vi "ModRegistered.vi"(8 "error in (no error)":errorcluster, 11 "JQMHStartup in":refnum<class "RQMHStartup.lvclass">) -> (0 "error out":errorcluster)   [LabVIEW 2024, in "RQMHStartup.lvclass"]
uses:
  RQMHStartup.lvclass
  Command.ctl
  RQMHStartup.lvclass/RQMHStartup.ctl
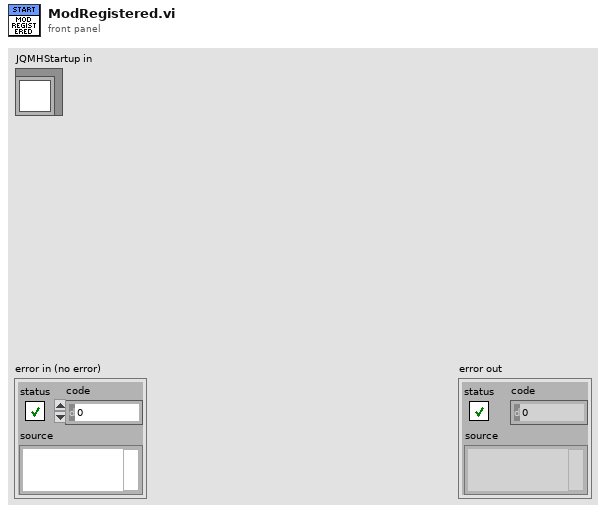
[diagram p1: front panel]
types:
  T1 = typedef "RQMHStartup.lvclass/Command.ctl" = enum16{"Default", "No Override", "Error", "ACK Created", "ACK Mod Reg", "ACK Caller Reg"}
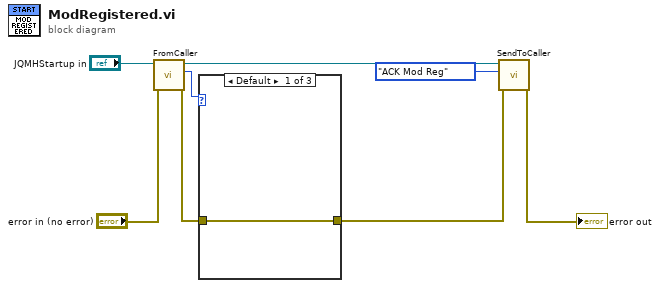
[diagram p0: block diagram]
diagram:
  n1 = call "FromCaller.vi"("error in (no error)"="error in (no error)", "JQMHStartup in"="JQMHStartup in") -> ("error out"=w5:errorcluster, "Command"=w6:T1, "JQMHStartup out"=w3:refnum<class "RQMHStartup.lvclass">)  [unwired: 6 in, 1 out]
  n2 = case shown="Default" w6 {
    tunnel: [w9 w10 w11] -> w1
    tunnel: w5 -> [w9 w10 w11]
    frame Default {
    }
    frame "Error" {
    }
    frame "ACK Caller Reg" {
    }
  }
  n3 = call "SendToCaller.vi"("error in (no error)"=w1, "Command"=Command."ACK Mod Reg", "JQMHStartup in"=w3) -> ("error out"=→"error out":errorcluster)  [unwired: 7 in, 1 out]
